vi "uTransport_Destroy.vi"(8 "error in (no error)":errorcluster, 11 "uClient_Publisher in":refnum<class "uClient_Publisher.lvclass">) -> (0 "error out":errorcluster)   [LabVIEW 2023, in "uLib.lvlib" / "uClient_Publisher.lvclass"]
uses:
  uClient_Publisher.lvclass
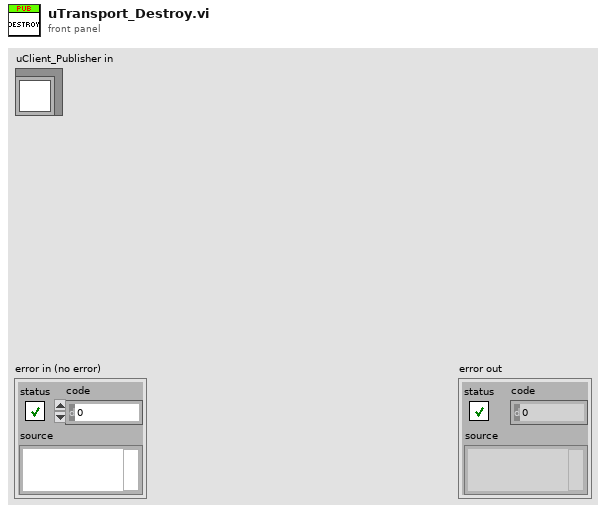
[diagram p1: front panel]
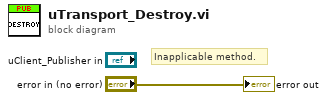
[diagram p0: block diagram]
diagram:
  # "Inapplicable method."
  "error out" <- "error in (no error)"
